vi "rqcBob Device Selector.vi"(8 "error in":errorcluster, 10 "Compatible Devices List":string[][](array[string])) -> (0 "error out":errorcluster, 1 "Device":string, 2 "Resource Name":string)   [LabVIEW 2018, in "rqcBob.lvclass"]
uses:
  rqcBob.lvclass
  <vilib>/Utility/error.llb/Error Cluster From Error Code.vi
  <vilib>/ErrorRing/Error Ring.xnode
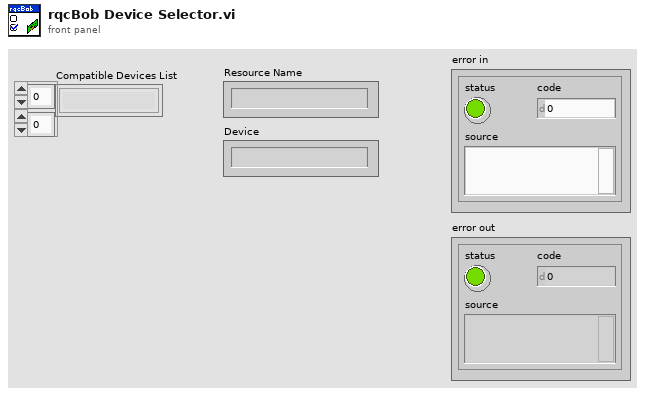
[diagram p1: front panel]
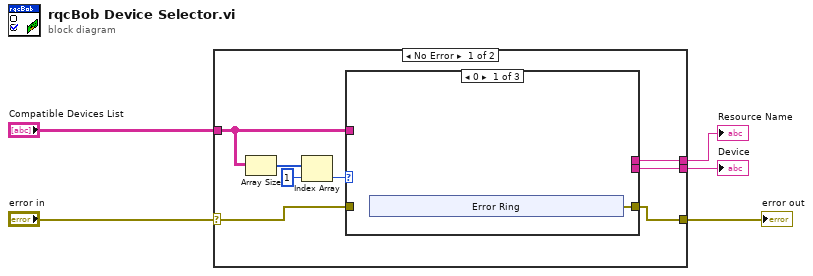
[diagram p0: block diagram]
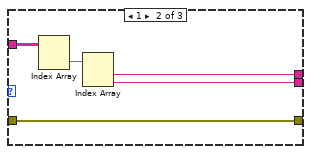
[diagram p2: hidden frame]
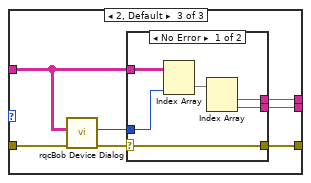
[diagram p3: hidden frame]
diagram:
  n1 = case shown="No Error" "error in" {
    selector: "error in" -> [w10 w38]
    tunnel: [w9 w38] -> w4
    tunnel: "Compatible Devices List" -> [w8 _]
    tunnel: [w7 _] -> w2
    tunnel: [w6 _] -> w1
    frame No Error {
      n2 = Array Size(array=w8) -> (size(s)=w13:i32[])
      n3 = Index Array(array=w13, index=1) -> (element=w11:i32)
      n4 = case shown="0" w11 {
        tunnel: w10 -> [_ w23 w30]
        tunnel: [w14 w23 w24] -> w9
        tunnel: w8 -> [_ w22 w28]
        tunnel: [_ w20 w26] -> w7
        tunnel: [_ w19 w25] -> w6
        frame 0 {
          n5 = xnode "Error Ring"() -> ("error out"=w14:errorcluster)
        }
        frame 1 {
          n6 = Index Array(array=w22) -> (element=w21:string[])  [unwired: 2 in]
          n7 = Index Array(array=w21) -> (element #1=w20:string, element #2=w19:string)  [unwired: 2 in]
        }
        frame 2, Default {
          n8 = call "rqcBob Device Dialog.vi"("error in"=w30, "Compatible Devices List"=w28) -> ("error out"=w29:errorcluster, "Device Index"=w27:i32)  [unwired: 8 in]
          n9 = case shown="No Error" w29 {
            selector: w29 -> [w31 w37]
            tunnel: w28 -> [w36 _]
            tunnel: w27 -> [w35 _]
            tunnel: [w33 _] -> w26
            tunnel: [w32 _] -> w25
            tunnel: [w31 w37] -> w24
            frame No Error {
              n10 = Index Array(array=w36, index (col)=w35) -> (element=w34:string[])  [unwired: 1 in]
              n11 = Index Array(array=w34) -> (element #1=w33:string, element #2=w32:string)  [unwired: 2 in]
            }
            frame Error {
            }
          }
        }
      }
    }
    frame Error {
    }
  }
  "error out" <- w4
  "Resource Name" <- w2
  "Device" <- w1
